vi "[FPGA] DeltaSig Main V4.vi"() -> ()   [LabVIEW 2015]
doc: "This VI provides a template for customizing a waveform acquisition using delta-sigma based NI C Series analog input smodules."
uses:
  <vilib>/LabVIEW Targets/FPGA/cRIO/shared/nicrio_ModuleControls/nicrio_cRIO-9234_ConfigModeRing.ctl
  <vilib>/rvi/Emulation/niFpgaGetClockAttributes.vi
  <vilib>/rvi/Emulation/niFpgaSctlEmulationGetInTimedLoop.vi
  <vilib>/rvi/Emulation/niFpgaEmulationReportErrorSimple.vi
  <vilib>/LabVIEW Targets/FPGA/cRIO/shared/nicrio_DsaDataRateApi/_nicrio_9234GetDataRate131.vi
  <vilib>/rvi/Emulation/niFpgaProcessEmulError.vi
  <vilib>/rvi/eio/common/nirviEmuTemplatePropertySet_errors.vi
  <vilib>/rvi/eio/common/nirviEmuTemplateMethod_errors.vi
  <vilib>/rvi/interface/RandomDataEmulation/niFpgaRandomDataHandleErrors.vi
  <vilib>/rvi/Emulation/niFpgaCriticalErrorInLSC.vi
  <vilib>/eio/EIOPropertyNode/EIOPropertyNode.xnode
  <vilib>/LabVIEW Targets/FPGA/cRIO/shared/nicrio_ModuleControls/nicrio_cRIO-9234_DataRatesRing2.ctl
  <vilib>/eio/EIONode/EIONode.xnode
  <vilib>/rvi/DataTransferAndStorage/Container/XNode/niFpgaContainer.xnode
  <vilib>/rvi/interface/RandomDataEmulation/nirviRandomDataFpgaReadWriteTemplate.vi
  <vilib>/rvi/eio/common/nirviEmuTemplatePropertyGet_errors.vi
  <vilib>/rvi/eio/common/nirviEmuTemplatePropertyGet_noerrors.vi
  <vilib>/rvi/eio/common/nirviEmuTemplatePropertySet_noerrors.vi
panel:
  in  "Array Input Config":T1[](array[typedef])=[0, 0, 0, 0, 0, 0, 0, 0] items=["AC Coupled", "DC Coupled", "IEPE AC Coupled"]
  out "oclk freq":u32
  out "oclk div":u32
  out "oclk mult":u32
  in  "data rate (S/s)":u32
  in  "Chan Scale Array":sgl[](array[numeric])=[0.0, 0.0, 0.0, 0.0, 0.0, 0.0, 0.0, 0.0, 0.0, 0.0, 0.0, 0.0, 0.0, 0.0, 0.0, 0.0, 0.0, 0.0, 0.0, 0.0, 0.0, 0.0, 0.0, 0.0, 0.0, 0.0, 0.0, 0.0, 0.0, 0.0, 0.0, 0.0, 0.0, 0.0, 0.0, 0.0, 0.0, 0.0, 0.0, 0.0]
  out "Chan Count":bool
  out "Acq Loop Ticks":u32
  out "FPGA Error":errorcluster
  out "Module Underflow":bool
  out "Finished":bool
  in  "Number of Channels":i32=8
  in  "Samps per Chan [Finite]":i32=5120
  out "First Read":bool
  in  "Acquisition Type":enum16{"Finite Samples", "Continuous Samples"}(ring)
  out "DMA FIFO Full":bool
  in  "stop":bool
  # "Array size fixed at 40\nelements but may be \nexpanded if needed"
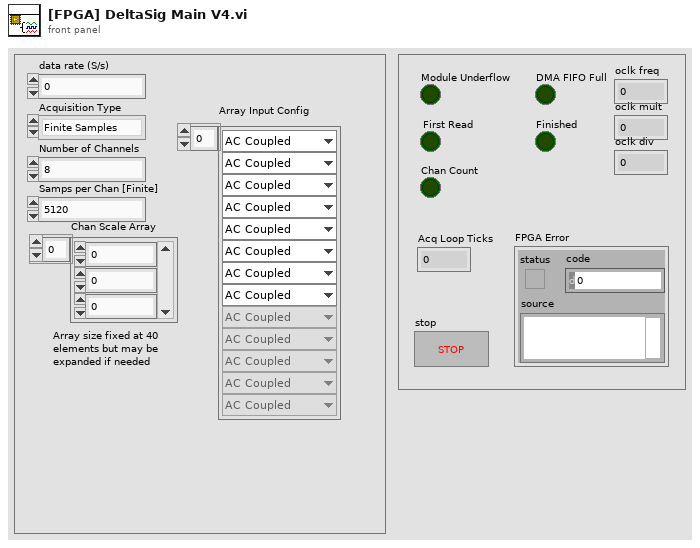
[diagram p1: front panel]
types:
  T1 = typedef "nicrio_cRIO-9234_ConfigModeRing.ctl" = u8
  T2 = typedef "nicrio_cRIO-9234_DataRatesRing2.ctl" = u8
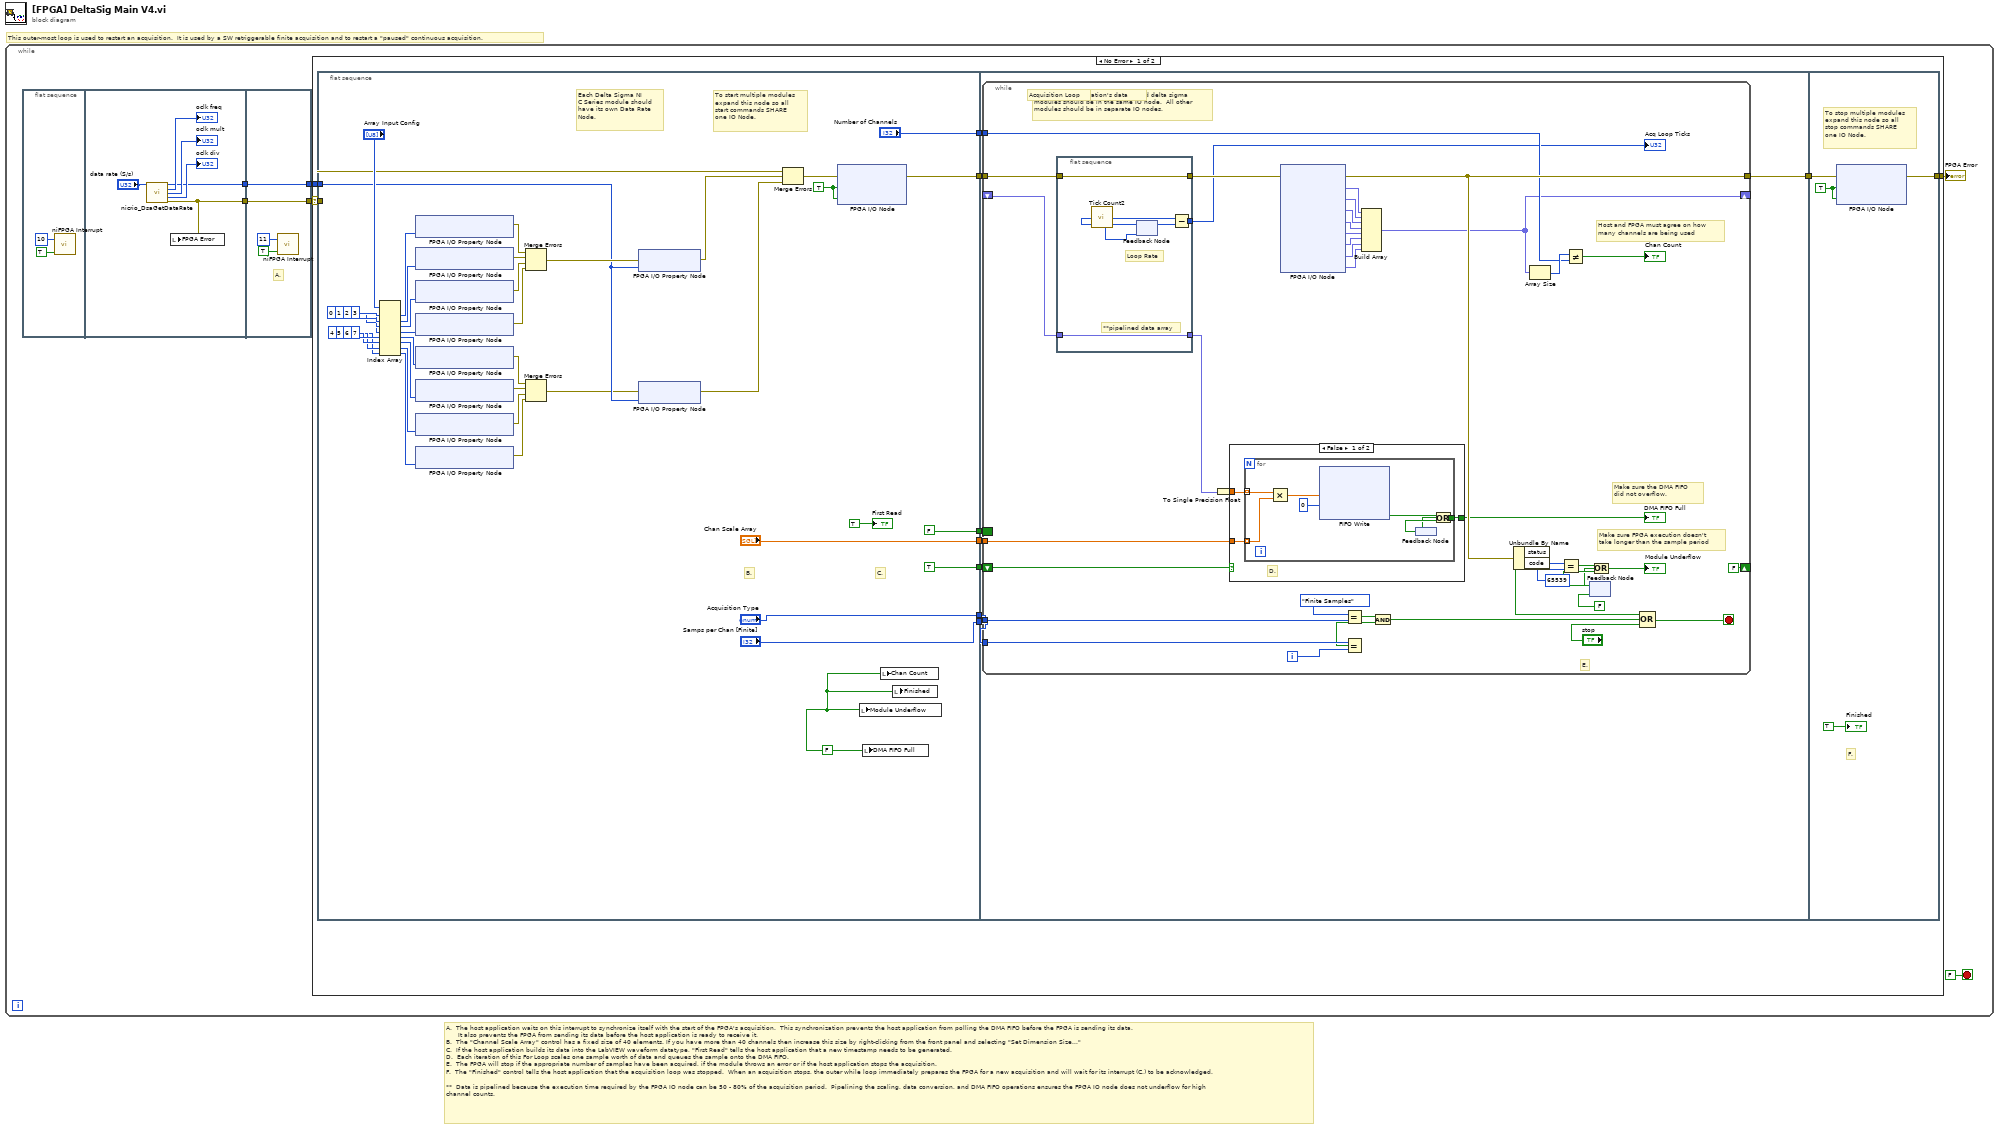
[diagram p0: block diagram]
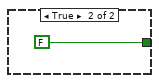
[diagram p2: hidden frame]
diagram:
  # "A.  The host application waits on this interrupt to synchronize itself with the start of the FPGA's acquisition.  This synchronization prevents the host application from polling the DMA FIFO before the FPGA is sending its data.\n      It also prevents the FPGA from sending its data before the host application is ready to receive it.\nB.  The \"Channel Scale Array\" control has a fixed size of 40 elements. If you have more than 40 channels then increase this size by right-clicking from the front panel and selecting \"Set Dimension Size...\"\nC.  If the host application builds its data into the LabVIEW waveform datatype, \"First Read\" tells the host application that a new timestamp needs to be generated.\nD.  Each iteration of this For Loop scales one sample worth of data and queues the sample onto the DMA FIFO.  \nE.  The FPGA will stop if the appropriate number of samples have been acquired, if the module throws an error or if the host application stops the acquisition.  \nF.  The \"Finished\" control tells the host application that the acquisition loop was stopped.  When an acquisition stops, the outer while loop immediately prepares the FPGA for a new acquisition and will wait for its interrupt (C.) to be acknowledged.\n\n**  Data is pipelined because the execution time required by the FPGA IO node can be 50 - 80% of the acquisition period.  Pipelining the scaling, data conversion, and DMA FIFO operations ensures the FPGA IO node does not underflow for high\nchannel counts."
  # "This outer-most loop is used to restart an acquisition.  It is used by a SW retriggerable finite acquisition and to restart a \"paused\" continuous acquisition."
  n1 = while {
    stop <- FALSE stop-if-true
    n2 = flat-sequence {
      tunnel: [w10] -> w2
      tunnel: [w11] -> w1
      tunnel: [w18] -> w3
      tunnel: [w15] -> w4
      tunnel: w2 -> [w15]
      tunnel: w1 -> [w18]
      frame #0 {
        n3 = call <vilib>:"niFPGA Interrupt.vi"("Wait Until Cleared (F)"=TRUE ("Wait Until Cleared"), "IRQ Number (0)"=u8 10 ("IRQ Number")) -> ()  [unwired: 1 in]
      }
      frame #1 {
        n4 = call-poly <vilib>:"nicrio_DsaGetDataRate.vi"("data rate (S/s)"="data rate (S/s)") -> ("data rate"=w11:T2, "oclk freq"=→"oclk freq":u32, "oclk mult"=→"oclk mult":u32, "oclk div"=→"oclk div":u32, "error out"=w10:errorcluster)  [unwired: 10 in]
        n5 = local write "FPGA Error"(w10) -> ()
      }
      frame #2 {
        # "A."
        n6 = call <vilib>:"niFPGA Interrupt.vi"("Wait Until Cleared (F)"=TRUE ("Wait Until Cleared"), "IRQ Number (0)"=u8 11 ("IRQ Number")) -> ()  [unwired: 1 in]
      }
    }
    n7 = case shown="No Error" w4 {
      selector: w4 -> [w19 w139]
      tunnel: [w21 w139] -> w5
      tunnel: w3 -> [w20 _]
      frame No Error {
        n8 = flat-sequence {
          tunnel: [w71] -> w29
          tunnel: ["Chan Scale Array"] -> w28
          tunnel: ["Acquisition Type"] -> w27
          tunnel: ["Samps per Chan [Finite]"] -> w26
          tunnel: ["Number of Channels"] -> w25
          tunnel: [TRUE ("t")] -> w24
          tunnel: [FALSE] -> w23
          tunnel: w20 -> [w48]
          tunnel: w19 -> [w42]
          tunnel: w29 -> [w78]
          tunnel: w28 -> [w77]
          tunnel: w27 -> [w75]
          tunnel: w26 -> [w74]
          tunnel: w25 -> [w79]
          tunnel: w24 -> [w76]
          tunnel: [w73] -> w22
          tunnel: w23 -> [w72]
          tunnel: w22 -> [w137]
          tunnel: [w136] -> w21
          frame #0 {
            w69 = FALSE ("Module Underflow")
            w30 = TRUE ("Mod1/Start")
            # "To start multiple modules\nexpand this node so all\nstart commands SHARE\none IO Node."
            # "C."
            # "B."
            # "Each Delta Sigma NI \nC Series module should \nhave its own Data Rate \nNode."
            n9 = Index Array(array="Array Input Config", index #1=0 ("index"), index #2=1 ("index"), index #3=2 ("index"), index #4=3 ("index"), index #5=4 ("index"), index #6=5 ("index"), index #7=6 ("index"), index #8=7 ("index")) -> (element #1=w61:T1, element #2=w60:T1, element #3=w59:T1, element #4=w58:T1, element #5=w38:T1, element #6=w37:T1, element #7=w36:T1, element #8=w35:T1)
            n10 = xnode "FPGA I/O Property Node"("Input Configuration"=w61) -> ("error out"=w54:errorcluster)  [unwired: 2 in, 1 out]
            n11 = xnode "FPGA I/O Property Node"("Input Configuration"=w60) -> ("error out"=w53:errorcluster)  [unwired: 2 in, 1 out]
            n12 = xnode "FPGA I/O Property Node"("Input Configuration"=w59) -> ("error out"=w52:errorcluster)  [unwired: 2 in, 1 out]
            n13 = xnode "FPGA I/O Property Node"("Input Configuration"=w58) -> ("error out"=w51:errorcluster)  [unwired: 2 in, 1 out]
            n14 = xnode "FPGA I/O Property Node"("Input Configuration"=w38) -> ("error out"=w47:errorcluster)  [unwired: 2 in, 1 out]
            n15 = xnode "FPGA I/O Property Node"("Input Configuration"=w37) -> ("error out"=w46:errorcluster)  [unwired: 2 in, 1 out]
            n16 = xnode "FPGA I/O Property Node"("Input Configuration"=w36) -> ("error out"=w45:errorcluster)  [unwired: 2 in, 1 out]
            n17 = xnode "FPGA I/O Property Node"("Input Configuration"=w35) -> ("error out"=w44:errorcluster)  [unwired: 2 in, 1 out]
            n18 = Merge Errors(w54, w53, w52, w51) -> (w50:errorcluster)
            n19 = Merge Errors(w47, w46, w45, w44) -> (w43:errorcluster)
            n20 = xnode "FPGA I/O Property Node"("error in"=w50, "Data Rate"=w48) -> ("error out"=w40:errorcluster)  [unwired: 1 in, 1 out]
            n21 = xnode "FPGA I/O Property Node"("error in"=w43, "Data Rate"=w48) -> ("error out"=w39:errorcluster)  [unwired: 1 in, 1 out]
            n22 = Merge Errors(w42, w40, w39) -> (w41:errorcluster)
            n23 = xnode "FPGA I/O Node"("error in"=w41, "Mod1/Start"=w30, "Mod2/Start"=w30) -> ("error out"=w71:errorcluster)  [unwired: 2 in, 2 out]
            n24 = local write "Module Underflow"(w69) -> ()
            n25 = local write "DMA FIFO Full"(w69) -> ()
            n26 = local write "Chan Count"(w69) -> ()
            n27 = local write "Finished"(w69) -> ()
            "First Read" <- TRUE ("First Read")
          }
          frame #1 {
            n28 = while {
              tunnel: w78 -> [w107]
              tunnel: [w112] -> w73
              tunnel: w75 -> [w114]
              tunnel: w74 -> [w113]
              shift-right: [w87] -> _
              shift-left: _ -> [w100]
              tunnel: w79 -> [w109]
              tunnel: w77 -> [w101]
              shift-right: [FALSE ("t")] -> _
              shift-left: w76 -> [w99]
              border: w72 -> [_]
              i -> [w97]
              stop <- w84 stop-if-true
              # "Add channels here.  All synchronized delta sigma\nmodules should be in the same IO node.  All other\nmodules should be in separate IO nodes."
              # "Do not DMA first iteration's data"
              # "Acquisition Loop"
              # "E."
              # "Host and FPGA must agree on how \nmany channels are being used"
              # "Make sure the DMA FIFO\ndid not overflow."
              # "Make sure FPGA execution doesn't\ntake longer than the sample period"
              n29 = flat-sequence {
                tunnel: [w123] -> w106
                tunnel: w107 -> [w123]
                tunnel: [w120] -> w105
                tunnel: w100 -> [w119]
                tunnel: [w119] -> w86
                frame #0 {
                  # "**pipelined data array"
                  # "Loop Rate"
                  n30 = call "Tick Count2"() -> ("Tick Count(Ticks)"=w122:u32)
                  n31 = feedback-in #1(w122) -> ()
                  n32 = feedback #1(w122) -> (w121:u32)
                  n33 = Subtract(x=w122, y=w121) -> (x-y=w120:u32)
                }
              }
              n34 = To Single Precision Float(number=w86) -> (single precision float=w85:sgl[])
              n35 = case shown="False" w99 {
                tunnel: [w126 FALSE] -> w111
                tunnel: w101 -> [w125 _]
                tunnel: w85 -> [w124 _]
                frame False {
                  # "D."
                  n36 = for {
                    tunnel: [w131] -> w126
                    tunnel: w124 -> [w129] mode=indexing
                    tunnel: w125 -> [w128] mode=indexing
                    n37 = Multiply(x=w129, y=w128) -> (x*y=w127:sgl)
                    n38 = xnode ("FIFO Write")("Element"=w127, "Timeout"=0) -> ("Timed Out?"=w133:bool)  [unwired: 1 in, 1 out]
                    n39 = feedback #2() -> (w132:bool)
                    n40 = Or(x=w133, y=w132) -> (x .or. y?=w131:bool)
                    n41 = feedback-in #2(w131) -> ()
                  }
                }
                frame True {
                }
              }
              "DMA FIFO Full" <- w111
              n42 = xnode "FPGA I/O Node"("error in"=w106) -> ("error out"=w112:errorcluster, "Mod1/AI0"=w104:fxp<+/-,24,4>, "Mod1/AI1"=w96:fxp<+/-,24,4>, "Mod1/AI2"=w103:fxp<+/-,24,4>, "Mod1/AI3"=w102:fxp<+/-,24,4>, "Mod2/AI0"=w83:fxp<+/-,24,4>, "Mod2/AI1"=w82:fxp<+/-,24,4>, "Mod2/AI2"=w81:fxp<+/-,24,4>, "Mod2/AI3"=w80:fxp<+/-,24,4>)  [unwired: 8 in, 8 out]
              n43 = Equal?(x=enum16{"Finite Samples", "Continuous Samples"}."Finite Samples" ("y"), y=w114) -> (x = y?=w90:bool)
              n44 = Equal?(x=w113, y=w97) -> (x = y?=w89:bool)
              n45 = Build Array(w104, w96, w103, w102, w83, w82, w81, w80) -> (w87:fxp<+/-,24,4>[])
              n46 = And(x=w90, y=w89) -> (x .and. y?=w88:bool)
              n47 = Unbundle By Name(w112) -> ("status"=w95:bool, "code"=w115:i32)
              n48 = Array Size(array=w87) -> (size(s)=w110:i32)
              n49 = Equal?(x=w115, y=65539) -> (x = y?=w92:bool)
              n50 = Not Equal?(x=w110, y=w109) -> (x != y?=→"Chan Count":bool)
              n51 = feedback #3(FALSE) -> (w94:bool)
              n52 = Or(x=w92, y=w94) -> (x .or. y?=w91:bool)
              "Module Underflow" <- w91
              n53 = feedback-in #3(w91) -> ()
              n54 = Compound Arithmetic op=OR(w95, w88, "stop") -> (w84:bool)
              "Acq Loop Ticks" <- w105
            }
          }
          frame #2 {
            w135 = TRUE ("Mod1/Stop")
            # "To stop multiple modules\nexpand this node so all\nstop commands SHARE\none IO Node."
            # "F."
            n55 = xnode "FPGA I/O Node"("error in"=w137, "Mod1/Stop"=w135, "Mod2/Stop"=w135) -> ("error out"=w136:errorcluster)  [unwired: 2 in, 2 out]
            "Finished" <- TRUE ("Finished")
          }
        }
      }
      frame Error {
      }
    }
    "FPGA Error" <- w5
  }
